vi "GetSet-ProductConfiguration.vi"(0 "Filepath":path, 5 "Product Configuration In":string[](array[string]), 7 "Read/Write":enum16{"Read", "Write"}(ring), 11 "Error In":errorcluster) -> (4 "Product Configuration Out":string[](array[string]), 15 "Error Out":errorcluster)   [LabVIEW 2015]
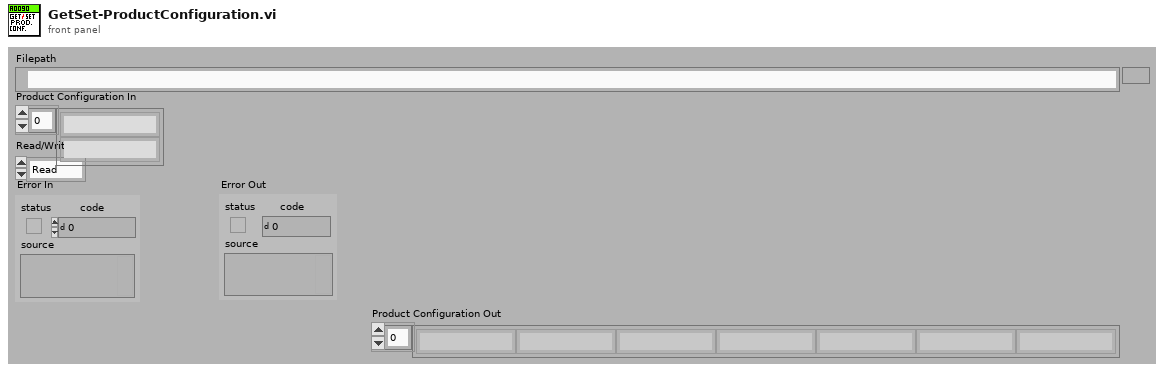
[diagram p1: front panel]
types:
  T1 = enum16{"read/write", "read-only", "write-only", "write-only (truncate)"}
  T2 = enum16{"open", "replace", "create", "open or create", "replace or create", "replace or create with confirmation"}
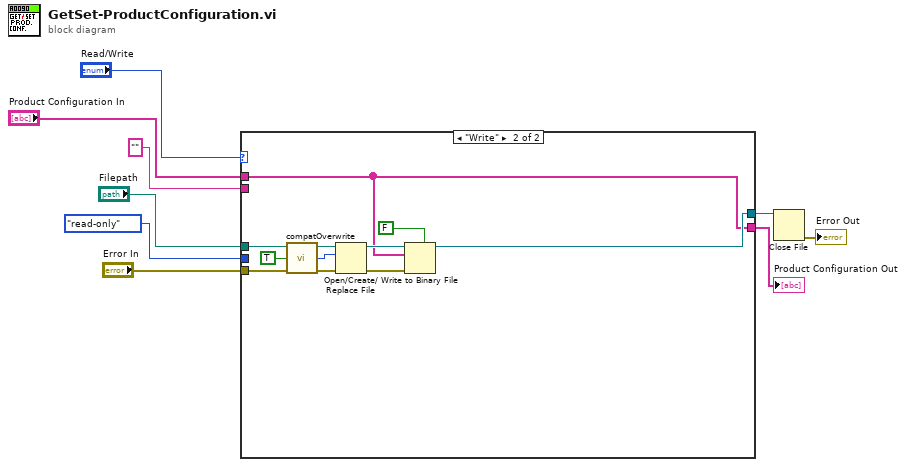
[diagram p0: block diagram]
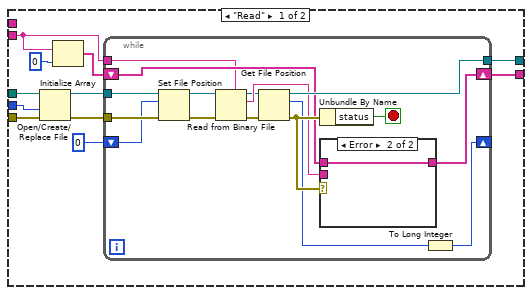
[diagram p2: hidden frame]
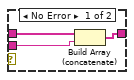
[diagram p3: hidden frame]
diagram:
  n1 = case shown="\"Write\"" "Read/Write" {
    tunnel: "Error In" -> [w20 w47]
    tunnel: "Filepath" -> [w17 w45]
    tunnel: [w16 w44] -> w9
    tunnel: T1."read-only" ("open mode (0)") -> [w15 _]
    tunnel: "Product Configuration In" -> [_ w43]
    tunnel: [w13 w43] -> w2
    tunnel: "" -> [w10 _]
    frame "Read" {
      n2 = Open/Create/Replace File(file path (use dialog)=w17, error in=w20, access (0:read/write)=w15) -> (refnum out=w19:refnum<file>, error out=w18:errorcluster)  [unwired: 3 in, 1 out]
      n3 = Initialize Array(w10, 0 ("dimension size")) -> (w12:string[])
      n4 = while {
        tunnel: w19 -> [w36]
        tunnel: w18 -> [w35]
        tunnel: [w34] -> w16
        shift-right: [w31] -> _
        shift-left: 0 ("offset") -> [w32]
        shift-right: [w27] -> w13
        shift-left: w12 -> [w28]
        tunnel: w10 -> [w26]
        stop <- w33 stop-if-true
        n5 = Set File Position(offset (in bytes) (0)=w32, refnum=w36, error in=w35) -> (refnum out=w25:refnum<file>, error out=w24:errorcluster)  [unwired: 1 in]
        n6 = Read from Binary File(5:w26, 8:w24, 11:w25) -> (0:w22:errorcluster, 2:w29:string, 3:w23:refnum<file>)  [unwired: 3 in, 1 out]
        n7 = Get File Position(4:w22, 7:w23) -> (0:w30:errorcluster, 2:w21:i64, 3:w34:refnum<file>)
        n8 = Unbundle By Name(w30) -> ("status"=w33:bool)
        n9 = case shown="Error" w30 {
          tunnel: w29 -> [w37 _]
          tunnel: [w39 w40] -> w27
          tunnel: w28 -> [w38 w40]
          frame No Error {
            n10 = Build Array (concatenate)(w38, w37) -> (w39:string[])
          }
          frame Error {
          }
        }
        n11 = To Long Integer(number=w21) -> (32bit integer=w31:i32)
      }
    }
    frame "Write" {
      n12 = call <vilib>:"compatOverwrite.vi"("overwrite (F)"=TRUE) -> ("overwrite?"=w42:T2)
      n13 = Open/Create/Replace File(file path (use dialog)=w45, error in=w47, operation (0:open)=w42) -> (refnum out=w49:refnum<file>, error out=w48:errorcluster)  [unwired: 3 in, 1 out]
      n14 = Write to Binary File(file (use dialog)=w49, data=w43, error in=w48, 5:FALSE ("prepend array or string size? (T)")) -> (refnum out=w44:refnum<file>)  [unwired: 2 in, 2 out]
    }
  }
  "Product Configuration Out" <- w2
  n15 = Close File(refnum=w9) -> (error out=→"Error Out":errorcluster)  [unwired: 1 in, 1 out]
